vi "String to Character Array.vi"(11 "input string":string="dsb") -> (3 "character array":string[](array[string]))   [LabVIEW 2022 SP3]
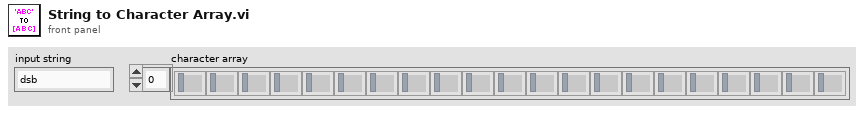
[diagram p1: front panel]
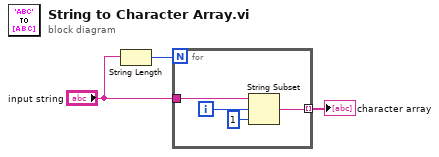
[diagram p0: block diagram]
diagram:
  n1 = String Length(string="input string") -> (length=w3:i32)
  n2 = for {
    N: w3 -> [_]
    tunnel: "input string" -> [w7]
    tunnel: [w4] -> w1 mode=indexing
    i -> [w6]
    n3 = String Subset(string=w7, offset (0)=w6, length (rest)=1 ("length (rest)")) -> (substring=w4:string)
  }
  "character array" <- w1
